vi "svx_Space Markers.vi"(9 "Z Scale Graph ref":refnum<vi>, 11 "markers in":dbl[](array[numeric])) -> (1 "Z Scale Graph ref out":refnum<vi>, 3 "markers out":dbl[](array[numeric]))   [LabVIEW 2017, in "SVX Waterfall Graph.xctl"]
uses:
  <vilib>/addons/_XControls/Waterfall Graph/SVX Waterfall Graph.xctl
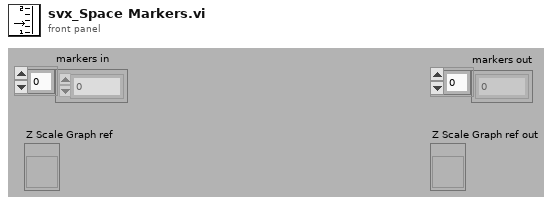
[diagram p1: front panel]
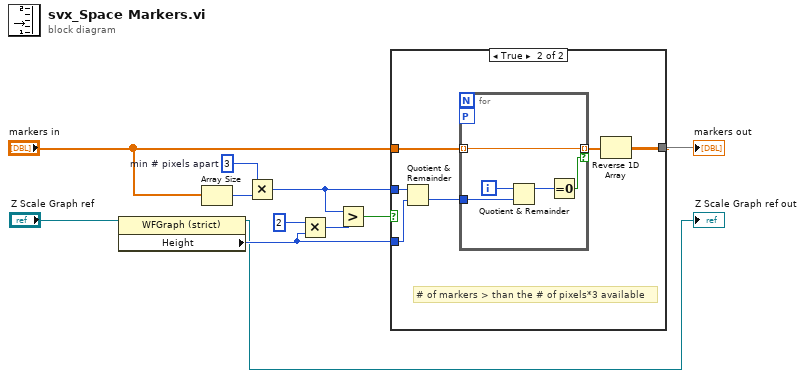
[diagram p0: block diagram]
diagram:
  w7 = u32 3  # min # pixels apart
  n1 = property on="Property Node" class="WFGraph (strict)"(reference="Z Scale Graph ref") -> (reference out=→"Z Scale Graph ref out":refnum<vi>, "Height"=w5:u32)  [unwired: 1 in, 1 out]
  n2 = Array Size(array="markers in") -> (size(s)=w8:i32)
  n3 = Multiply(x=w7, y=w8) -> (x*y=w6:u32)
  n4 = Multiply(x=u32 2 ("y"), y=w5) -> (x*y=w3:u32)
  n5 = Greater?(x=w6, y=w3) -> (0:w10:bool)
  n6 = case shown="True" w10 {
    tunnel: "markers in" -> [w12 w18]
    tunnel: [w12 w13] -> w11
    tunnel: w6 -> [_ w17]
    tunnel: w5 -> [_ w16]
    frame False {
      # "enough spacing for the markers"
    }
    frame True {
      # "# of markers > than the # of pixels*3 available"
      n7 = Quotient & Remainder(x=w17, y=w16) -> (floor(x/y)=w15:u32)  [unwired: 1 out]
      n8 = for {
        tunnel: w18 -> [w20] mode=indexing
        tunnel: w15 -> [w22]
        tunnel: [w20] -> w14 mode=indexing if=w19
        workers-P: _ -> [_]
        i -> [w23]
        n9 = Quotient & Remainder(x=w23, y=w22) -> (x-y*floor(x/y)=w21:u32)  [unwired: 1 out]
        n10 = Equal To 0?(x=w21) -> (x = 0?=w19:bool)
      }
      n11 = Reverse 1D Array(array=w14) -> (reversed array=w13:dbl[])
    }
  }
  "markers out" <- w11
